vi "Compile DIO.vi"(8 "error in (no error)":errorcluster, 11 "Device Item Ref in":T1 format="%.0x") -> (0 "error out":errorcluster, 2 "Initial DIO SPI CMDs":u64[](array[numeric]), 3 "Device Item Ref out":T1 format="%.0x")   [LabVIEW 2014, in "SLSC configuration System Explorer.lvlib"]
uses:
  SLSC configuration System Explorer.lvlib
  <vilib>/NI Veristand/Custom Device API/Custom Device Item Ref.ctl
  Shared/Constants.vi
  <vilib>/NI Veristand/Custom Device API/Get Item Property (U16).vi
  <vilib>/NI Veristand/Custom Device Tools/Custom Device Utility Library/Custom Device Utility Library.lvlib
  Shared/SLSC configuration Shared.lvlib
  <vilib>/NI Veristand/Custom Device API/Custom Device API.lvlib
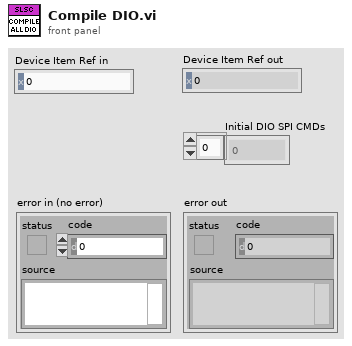
[diagram p1: front panel]
types:
  T1 = typedef "Custom Device API.lvlib/Custom Device Item Ref.ctl" = u64
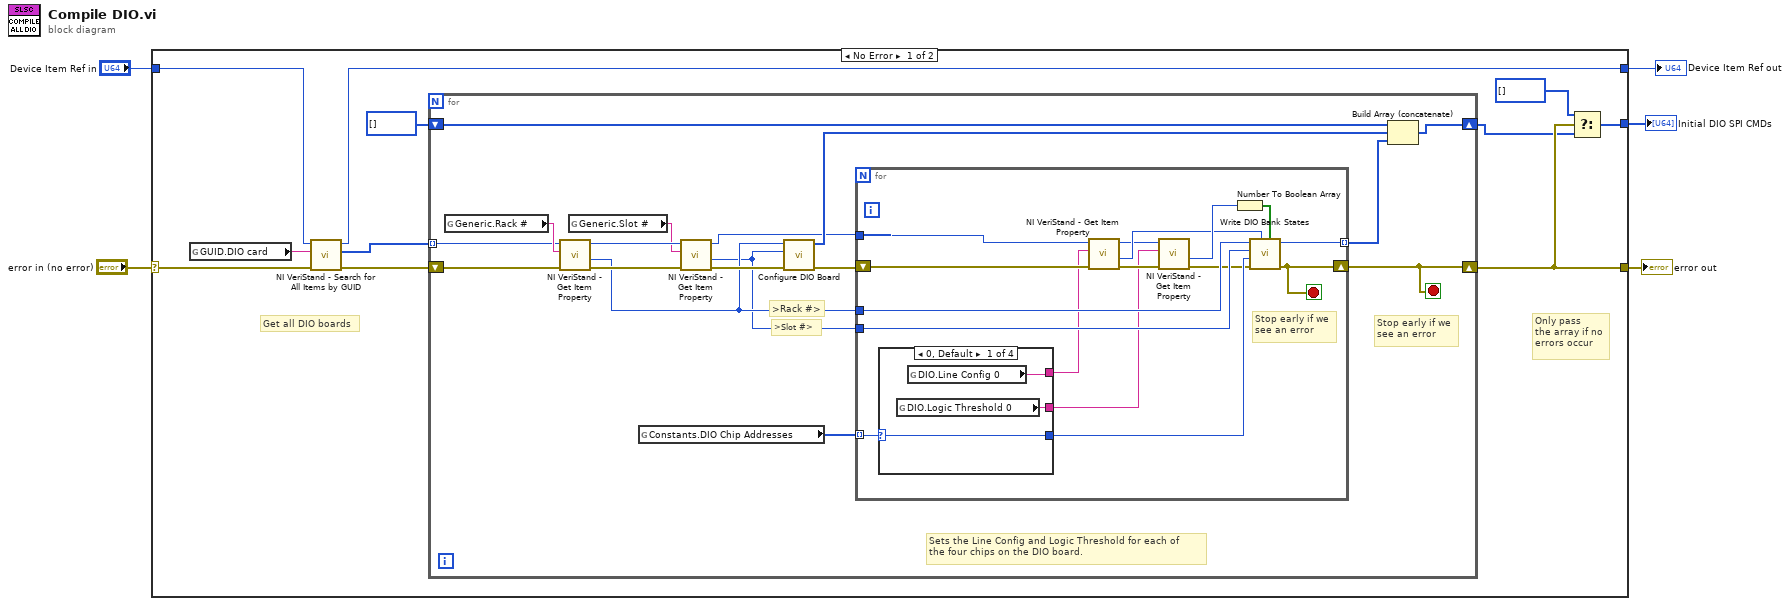
[diagram p0: block diagram]
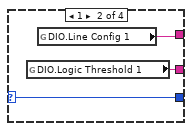
[diagram p2: hidden frame]
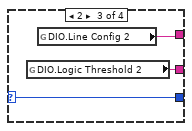
[diagram p3: hidden frame]
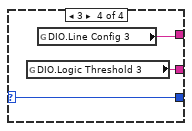
[diagram p4: hidden frame]
diagram:
  n1 = case shown="No Error" "error in (no error)" {
    selector: "error in (no error)" -> [w12 w63]
    tunnel: "Device Item Ref in" -> [w14 w62]
    tunnel: [w9 w63] -> w4
    tunnel: [w11 w62] -> w2
    tunnel: [w7 _] -> w1
    frame No Error {
      # "Only pass\nthe array if no\nerrors occur"
      # "Get all DIO boards"
      n2 = global read "Constants.vi" "GUID.DIO card"() -> (w16:string)
      n3 = call <vilib>:"NI VeriStand - Search for All Items by GUID.vi"("error in"=w12, "Item GUID"=w16, "Section Ref in"=w14) -> ("error out"=w13:errorcluster, "Item Refs"=w15:T1[], "Section Ref out"=w11:T1)  [unwired: 5 in, 1 out]
      n4 = for {
        shift-right: [w18] -> w9
        shift-left: w13 -> [w28]
        tunnel: w15 -> [w29] mode=indexing
        shift-right: [w17] -> w8
        shift-left: u64[] [] -> [w23]
        stop <- w18 stop-if-true
        # "Stop early if we\nsee an error"
        # "Sets the Line Config and Logic Threshold for each of\nthe four chips on the DIO board."
        # ">Slot #>"
        # ">Rack #>"
        n5 = global read "Constants.vi" "Generic.Rack #"() -> (w30:string)
        n6 = call-poly <vilib>:"NI VeriStand - Get Item Property.vi"("error in (no error)"=w28, "Property Name"=w30, "Item Ref in"=w29) -> ("error out"=w32:errorcluster, "Value"=w25:u16, "Item Ref out"=w33:T1)  [unwired: 5 in, 1 out]
        n7 = global read "Constants.vi" "Generic.Slot #"() -> (w31:string)
        n8 = global read "Constants.vi" "Constants.DIO Chip Addresses"() -> (w20:u8[])
        n9 = call-poly <vilib>:"NI VeriStand - Get Item Property.vi"("error in (no error)"=w32, "Property Name"=w31, "Item Ref in"=w33) -> ("error out"=w27:errorcluster, "Value"=w21:u16, "Item Ref out"=w22:T1)  [unwired: 5 in, 1 out]
        n10 = call "Configure DIO Board.vi"("error in (no error)"=w27, "Slot #"=w21, "Rack #"=w25) -> ("error out"=w19:errorcluster, "SPI FIFO Messages"=w26:u64[])  [unwired: 7 in]
        n11 = for {
          tunnel: w20 -> [w39] mode=indexing
          tunnel: w25 -> [w45]
          tunnel: w21 -> [w46]
          tunnel: [w49] -> w24 mode=indexing
          shift-right: [w34] -> w18
          shift-left: w19 -> [w48]
          tunnel: w22 -> [w47]
          stop <- w34 stop-if-true
          # "Stop early if we\nsee an error"
          n12 = case shown="0, Default" w39 {
            selector: w39 -> [w52 w55 w58 w61]
            tunnel: [w52 w55 w58 w61] -> w38
            tunnel: [w51 w54 w57 w60] -> w37
            tunnel: [w50 w53 w56 w59] -> w36
            frame 0, Default {
              n13 = global read "Constants.vi" "DIO.Logic Threshold 0"() -> (w50:string)
              n14 = global read "Constants.vi" "DIO.Line Config 0"() -> (w51:string)
            }
            frame 1 {
              n15 = global read "Constants.vi" "DIO.Logic Threshold 1"() -> (w53:string)
              n16 = global read "Constants.vi" "DIO.Line Config 1"() -> (w54:string)
            }
            frame 2 {
              n17 = global read "Constants.vi" "DIO.Logic Threshold 2"() -> (w56:string)
              n18 = global read "Constants.vi" "DIO.Line Config 2"() -> (w57:string)
            }
            frame 3 {
              n19 = global read "Constants.vi" "DIO.Logic Threshold 3"() -> (w59:string)
              n20 = global read "Constants.vi" "DIO.Line Config 3"() -> (w60:string)
            }
          }
          n21 = call-poly <vilib>:"NI VeriStand - Get Item Property.vi"("error in (no error)"=w48, "Property Name"=w37, "Item Ref in"=w47) -> ("error out"=w44:errorcluster, "Value"=w41:u16, "Item Ref out"=w40:T1)  [unwired: 5 in, 1 out]
          n22 = call-poly <vilib>:"NI VeriStand - Get Item Property.vi"("error in (no error)"=w44, "Property Name"=w36, "Item Ref in"=w40) -> ("error out"=w35:errorcluster, "Value"=w43:u16)  [unwired: 5 in, 2 out]
          n23 = Number To Boolean Array(number=w43) -> (Boolean array=w42:bool[])
          n24 = call "Write DIO Bank States.vi"("DIO Line Config"=w42, "Logic Threshold (%)"=w41, "error in (no error)"=w35, "Chip Address (A2 A1 A0)"=w38, "Slot #"=w46, "Rack #"=w45) -> ("error out"=w34:errorcluster, "FIFO SPI Message"=w49:u64)  [unwired: 3 in, 1 out]
        }
        n25 = Build Array (concatenate)(w23, w26, w24) -> (w17:u64[])
      }
      n26 = Select(t=u64[] [], s=w9, f=w8) -> (s? t:f=w7:u64[])
    }
    frame Error {
    }
  }
  "error out" <- w4
  "Device Item Ref out" <- w2
  "Initial DIO SPI CMDs" <- w1
